vi "Read startTime.vi"(8 "error in (no error)":errorcluster, 11 "PrimaryAttackerRole in":refnum<class "PrimaryAttackerRole.lvclass">) -> (0 "error out":errorcluster, 2 "startTime":timestamp, 3 "PrimaryAttackerRole out":refnum<class "PrimaryAttackerRole.lvclass">)   [LabVIEW 2023, in "PrimaryAttackerRole.lvclass"]
uses:
  PrimaryAttackerRole.lvclass
  PrimaryAttackerRole.lvclass/PrimaryAttackerRole.ctl
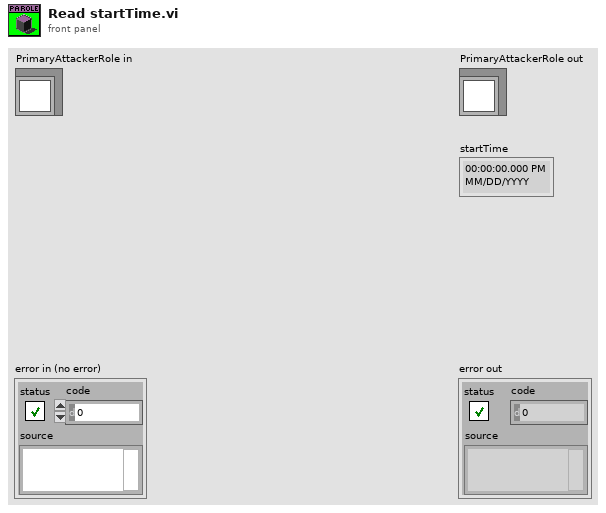
[diagram p1: front panel]
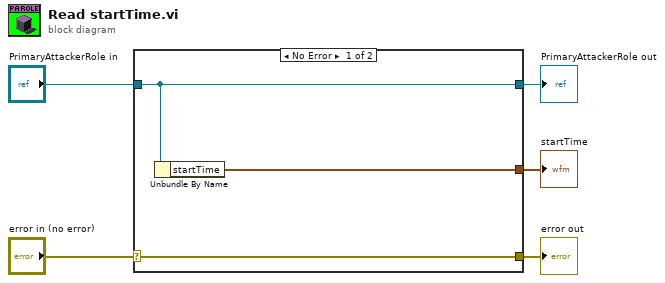
[diagram p0: block diagram]
diagram:
  n1 = case shown="No Error" "error in (no error)" {
    selector: "error in (no error)" -> [w8 w9]
    tunnel: [w8 w9] -> w4
    tunnel: [w7 w10] -> w2
    tunnel: "PrimaryAttackerRole in" -> [w7 w10]
    tunnel: [w6 _] -> w1
    frame No Error {
      n2 = Unbundle By Name(w7) -> ("startTime"=w6:timestamp)
    }
    frame Error {
    }
  }
  "error out" <- w4
  "PrimaryAttackerRole out" <- w2
  "startTime" <- w1
